vi "FTW-Message-Lossy-Multipart-Initialize.vi"(0 "FTW-Message-Lossy In":refnum<class "FTW-Message-Lossy.lvclass">, 1 "Queue":refnum<queue>, 5 "Message Parts":string[](array[string]), 11 "error in":errorcluster) -> (4 "FTW-Message-Lossy Out":refnum<class "FTW-Message-Lossy.lvclass">, 6 "overflow?":bool, 15 "error out":errorcluster)   [LabVIEW 2013, in "FTW-Message-Lossy.lvclass"]
uses:
  FTW-Message-Lossy.lvclass
  FTW-Message-Lossy.lvclass/FTW-Message-Lossy.ctl
panel:
  # "Inputs"
  # "Outputs"
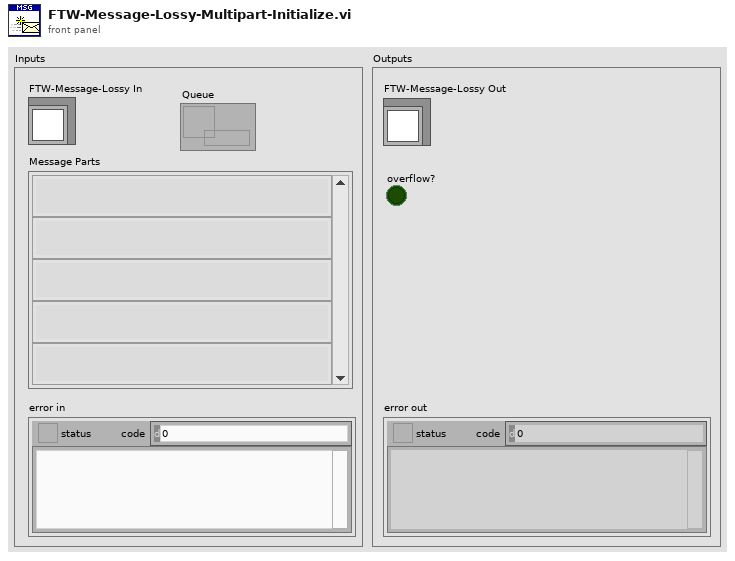
[diagram p1: front panel]
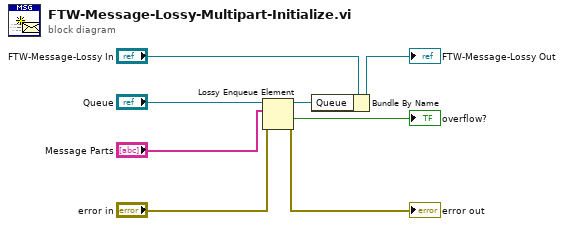
[diagram p0: block diagram]
diagram:
  n1 = Lossy Enqueue Element(queue="Queue", element="Message Parts", error in (no error)="error in") -> (queue out=w3:refnum<queue>, overflow?=→"overflow?":bool, error out=→"error out":errorcluster)  [unwired: 1 out]
  n2 = Bundle By Name(cluster="FTW-Message-Lossy In", "Queue"=w3) -> (→"FTW-Message-Lossy Out":refnum<class "FTW-Message-Lossy.lvclass">)
